vi "Ref Est.vi"(9 "touch":bool, 10 "IA State Input":T2) -> (1 "IA command":T1, 2 "IA State Output":T2)   [LabVIEW 2024, in "Referee.lvclass"]
uses:
  Referee.lvclass
  Vision_class/Old vision/SSL Detection Frame Simple Estimator Cameras VelCmd Folder/Core/AI Input.ctl
  Vision_class/Old vision/Controls/AI Robot.ctl
  Vision_class/Old vision/Controls/Functions Enum.ctl
  Controls/estimatives.ctl
  Vision_class/Old vision/Controls/AttackerStates.ctl
  Vision_class/Old vision/Controls/PathDests.ctl
  Vision_class/Old vision/Controls/PathDest.ctl
  Game_class/Navigation/VSSNavigation/VSSAttackerStates.ctl
  Robot_class/robotKickToStates.ctl
  Robot_class/roles.ctl
  <vilib>/Analysis/Matrix/Datatypes/RealMatrix.ctl
  Game_class/Navigation/driveMode.ctl
  Vision_class/Old vision/SSL Detection Frame Simple Estimator Cameras VelCmd Folder/Core/AI Ball.ctl
  Vision_class/Old vision/SSL Detection Frame Simple Estimator Cameras VelCmd Folder/Core/Field Size.ctl
  Vision_class/Old vision/SSL Detection Frame Simple Estimator Cameras VelCmd Folder/Core/AI Judge.ctl
  Communication_class/Paths/MessageAI_State Folder/Intel/Command Enum.ctl
  Vision_class/Old vision/SSL Detection Frame Simple Estimator Cameras VelCmd Folder/Util/Events/Events.ctl
  <vilib>/Analysis/Matrix/NI_Matrix.lvlib
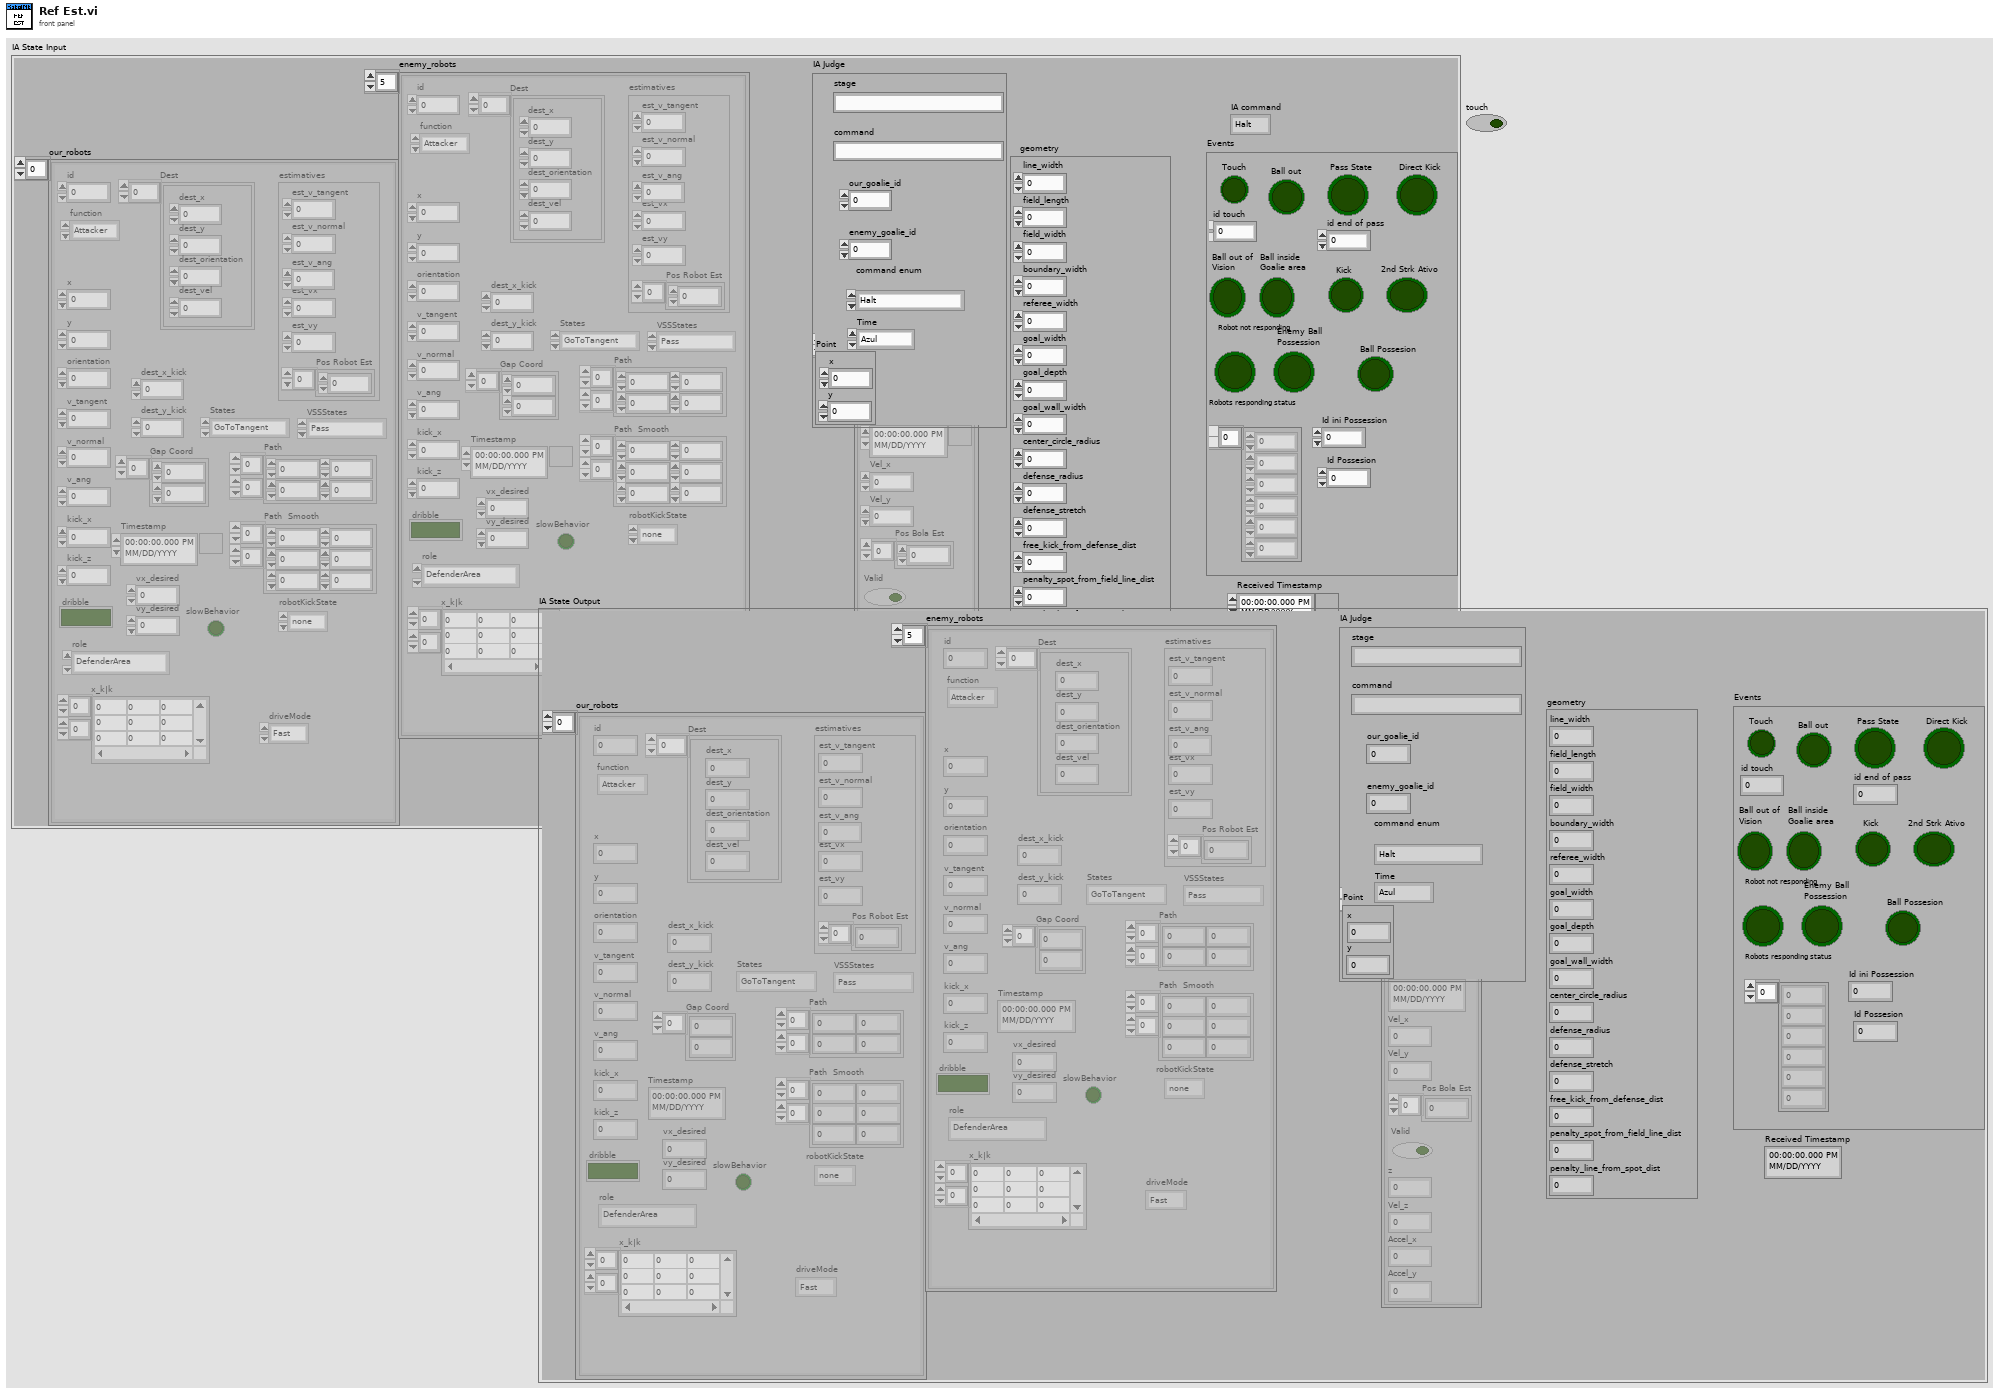
[diagram p1: front panel]
types:
  T1 = typedef "Command Enum.ctl" = enum16{"Halt", "Stop", "Force Start", "PKA Normal Start", "Prepare Kickoff Ally", "PKE Normal Start", "Prepare Kickoff Enemy", "Prepare Penalty Ally", "PPA Normal Start", "Prepare Penalty Enemy", "PPE Normal Start", "Direct Free Enemy", "Direct Free Ally", "Indirect Free Enemy", "Indirect Free Ally", "Timeout Enemy", "Timeout Ally", "Goal Enemy", "Goal Ally", "Ball Placement Enemy", "Ball Placement Ally", "Normal Half Time", "Extra Time Break", "Extra Half Time", "None", "Post Game", "S Normal Start"}
  T2 = typedef "AI Input.ctl" = cluster{"our_robots":T3[], "enemy_robots":T3[], "balls":T14[], "geometry":T15, "IA Judge":T16, "Received Timestamp":timestamp, "Events":T17}
  T3 = typedef "AI Robot.ctl" = cluster{"id":u32, "function":T4, "x":dbl, "y":dbl, "orientation":dbl, "v_tangent":dbl, "v_normal":dbl, "v_ang":dbl, "kick_x":dbl, "kick_z":dbl, "dribble":bool, "Timestamp":timestamp, "estimatives":T5, "dest_x_kick":dbl, "dest_y_kick":dbl, "Gap Coord":dbl[], "States":T6, "Path ":dbl[][], "Path  Smooth":dbl[][], "Dest":T7, "vx_desired":dbl, "vy_desired":dbl, "slowBehavior":bool, "VSSStates":T9, "robotKickState":T10, "role":T11, "x_k|k":T12, "driveMode":T13}
  T4 = typedef "Functions Enum.ctl" = enum16{"2nd Striker", "Attacker", "Goalie", "Defender", "Striker", "Goto 0", "Dummy", "Kicker", "ZigZag 0", "ZigZag 1", "ZigZag 2", "ZigZag 3", "ZigZag 4", "ZigZag 5", "ZigZag 6", "ZigZag 7", "ZigZag 8", ""}
  T5 = typedef "estimatives.ctl" = cluster{"est_v_tangent":dbl, "est_v_normal":dbl, "est_vx":dbl, "est_vy":dbl, "Pos Robot Est":dbl[], "est_v_ang":dbl}
  T6 = typedef "AttackerStates.ctl" = enum16{"Pass", "GoToTangent", "BallGetting", "GoToKick", ""}
  T7 = typedef "PathDests.ctl" = T8[]
  T8 = typedef "PathDest.ctl" = cluster{"dest_x":dbl, "dest_y":dbl, "dest_orientation":dbl, "dest_vel":dbl}
  T9 = typedef "VSSAttackerStates.ctl" = enum16{"Pass", "GoToTangent", "BallGetting", "GoToKick", "Rotate anti-clockwise", "Rotate Clockwise", ""}
  T10 = typedef "robotKickToStates.ctl" = enum16{"shootFromDirect", "avoidCollideBall", "goToBackBall", "none", "walk", "turn", "turnAntiClockWise", "turnClockwise", "oldKickToShoot", "oldKickToGoToBackBall", "shoot"}
  T11 = typedef "roles.ctl" = enum16{"SimpleBallPlacement", "BallPlacementAllyPasser", "BallPlacementAllyReceiver", "BallPlacementEnemy", "5Robots5th", "PassBestReceiver", "5Robots4th", "5Robots3rd", "5Robots2nd", "5Robots1st", "PassBestRobot", "WaitPass", "ABCThirdKicker", "ABCFirstKicker", "ABCSecondKicker", "Tabler", "TableFinalizer", "PrepareRollToPassRoller", "PrepareRollToPassReceiver", "SimplePassRoll", "SimplePassRollReceiver", "PenaltyDefense", "PreparePassReceiver 2", "PreparePassReceiver 1", "PassObserver", "Timeout", "Goto", "ZigZag", "None", "BallOutOfField", "DefenderArea", "Duelist", "AttackerStop", "FollowAttacker", "KeeperRole", "KickPenalty", "AttackerAimGoal", "AttackerBlock", "Marker", "Halt", "Shoot", "PassKicker", "PassReceiver", "TestRole", "PenaltyAttacker"}
  T12 = typedef "NI_Matrix.lvlib/RealMatrix.ctl" = dbl[][]
  T13 = typedef "driveMode.ctl" = enum16{"Fast", "SafeDrive"}
  T14 = typedef "AI Ball.ctl" = cluster{"x":dbl, "y":dbl, "timestamp":timestamp, "Vel_x":dbl, "Vel_y":dbl, "Pos Bola Est":dbl[], "Valid":bool, "z":dbl, "Vel_z":dbl, "Accel_x":dbl, "Accel_y":dbl}
  T15 = typedef "Field Size.ctl" = cluster{"line_width":u32, "field_length":u32, "field_width":u32, "boundary_width":u32, "referee_width":u32, "goal_width":u32, "goal_depth":u32, "goal_wall_width":u32, "center_circle_radius":u32, "defense_radius":u32, "defense_stretch":u32, "free_kick_from_defense_dist":u32, "penalty_spot_from_field_line_dist":u32, "penalty_line_from_spot_dist":u32}
  T16 = typedef "AI Judge.ctl" = cluster{"stage":string, "command":string, "our_goalie_id":dbl, "enemy_goalie_id":dbl, "command enum":T1, "Time":enum16{"Azul", "Amarelo"}, "Point":cluster{"x":sgl, "y":sgl}}
  T17 = typedef "Events.ctl" = cluster{"Touch":bool, "Ball out":bool, "id touch":dbl, "Ball out of \nVision":bool, "Ball inside \nGoalie area":bool, "Robot not responding":bool, "Robots responding status":dbl[], "Enemy Ball \nPossession":bool, "Pass State":bool, "id end of pass":dbl, "Kick":bool, "Id ini Possession":dbl, "Ball Possesion":bool, "Id Possesion":dbl, "Direct Kick":bool, "2nd Strk Ativo":bool}
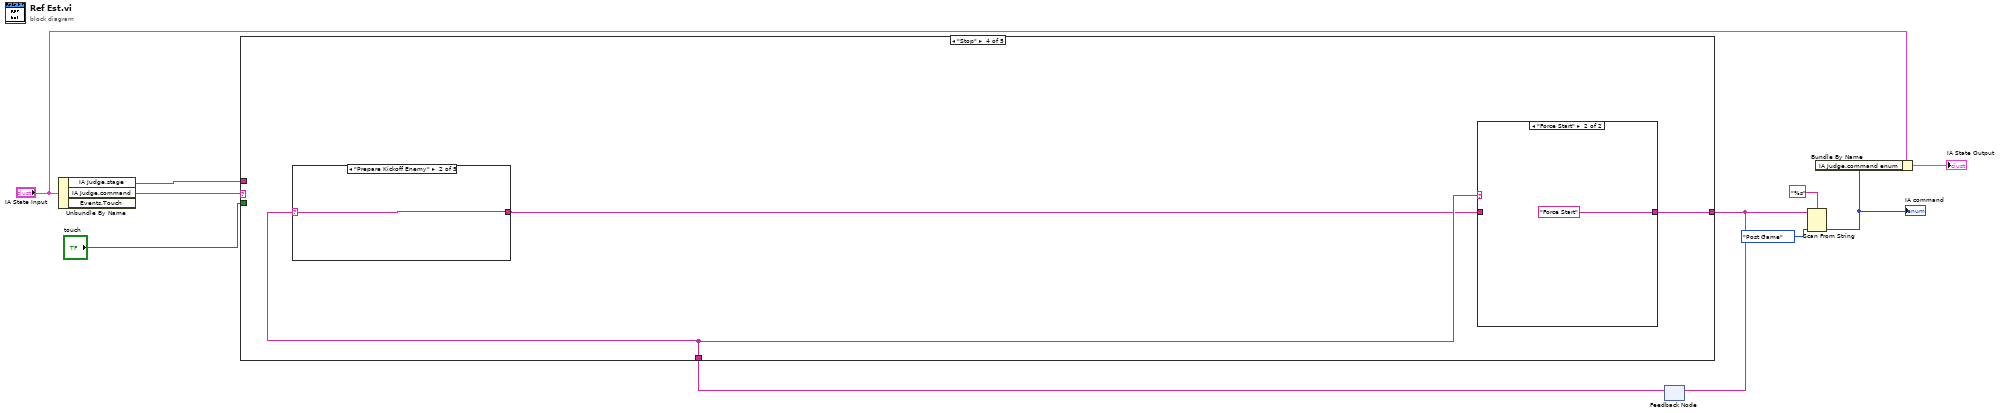
[diagram p0: block diagram]
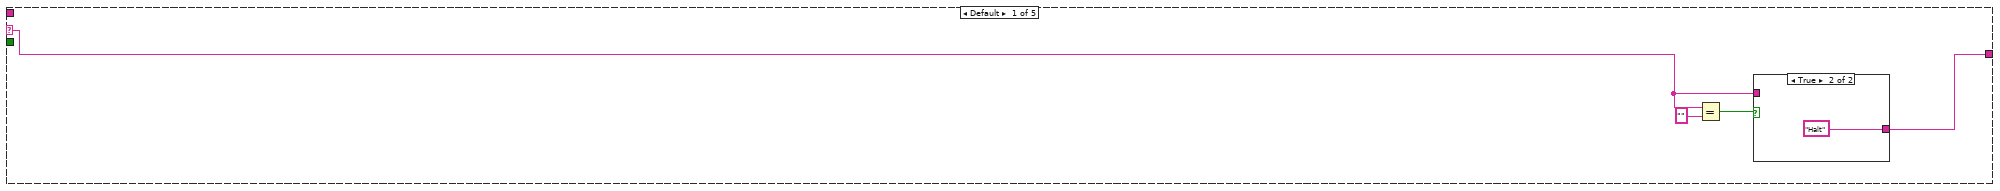
[diagram p2: hidden frame]
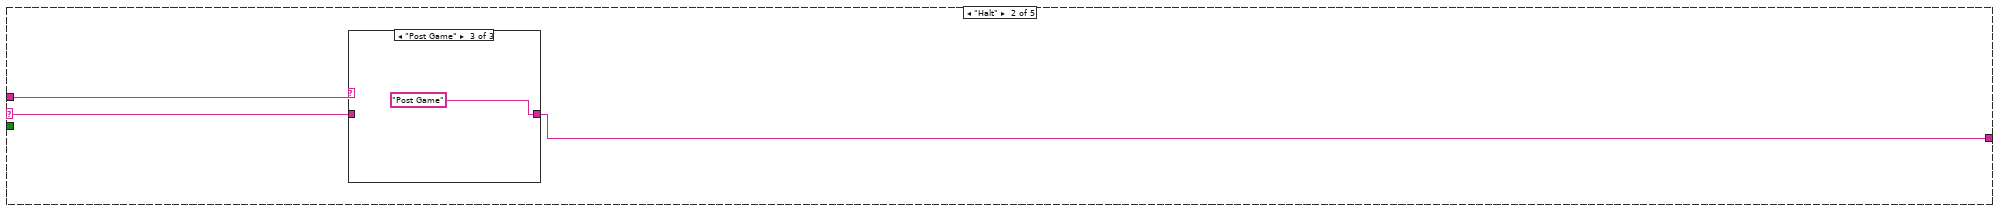
[diagram p4: hidden frame]
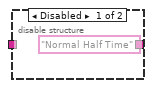
[diagram p7: hidden frame]
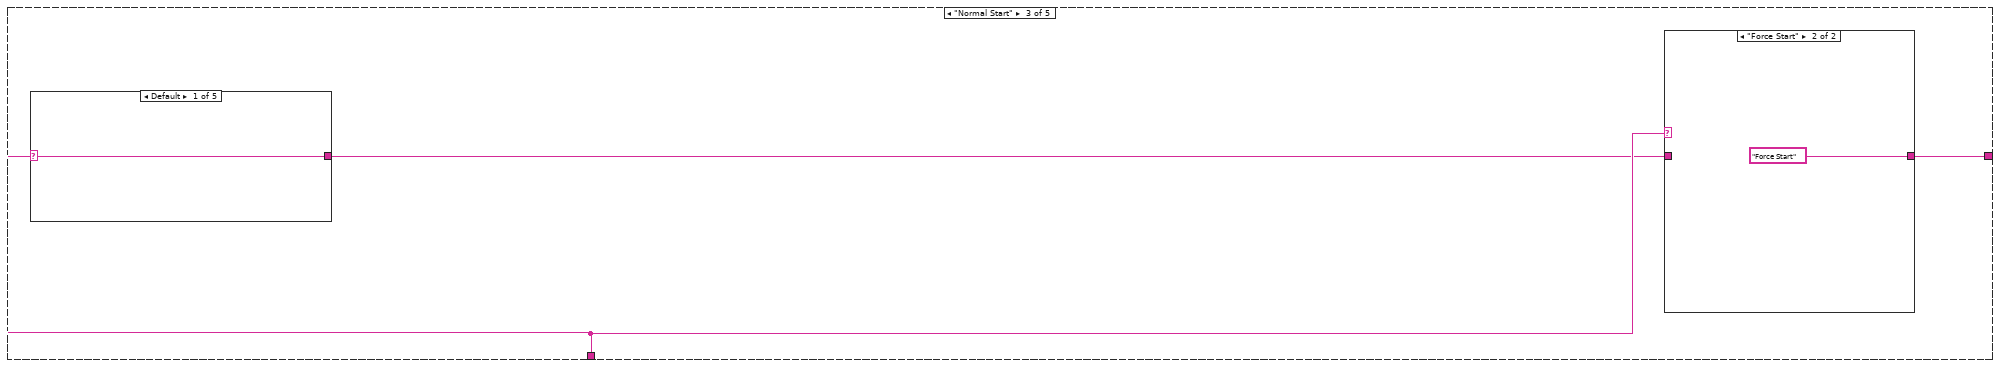
[diagram p8: hidden frame]
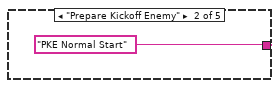
[diagram p10: hidden frame]
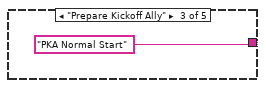
[diagram p11: hidden frame]
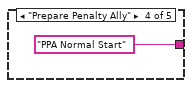
[diagram p12: hidden frame]
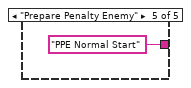
[diagram p13: hidden frame]
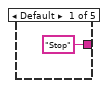
[diagram p15: hidden frame]
diagram:
  n1 = Unbundle By Name("IA State Input") -> ("IA Judge.stage"=w3:string, "IA Judge.command"=w10:string)  [unwired: 1 out]
  n2 = feedback #1() -> (w5:string)  [unwired: 1 in]
  n3 = case shown="\"Stop\"" w10 {
    selector: w10 -> [w11 w18 _ _ w46]
    tunnel: [w13 w17 w28 w38 w46] -> w4
    tunnel: w5 -> [_ _ w27 w37 _]
    tunnel: "touch" -> [_ _ _ _ _]
    tunnel: w3 -> [_ w19 _ _ _]
    frame Default {
      n4 = Equal?(x=w11, y="") -> (x = y?=w12:bool)
      n5 = case shown="True" w12 {
        tunnel: [w15 "Halt" ("y")] -> w13
        tunnel: w11 -> [w15 _]
        frame False {
        }
        frame True {
        }
      }
    }
    frame "Halt" {
      n6 = case shown="\"Post Game\"" w19 {
        tunnel: [w20 w22 "Post Game"] -> w17
        tunnel: w18 -> [w20 w21 _]
        frame Default {
        }
        frame "Normal Half Time" {
          n7 = disable-structure shown="Enabled" {
            disable-tunnel: ["Normal Half Time" w24] -> w22
            disable-tunnel: w21 -> [_ w24]
            frame Disabled {
            }
            frame Enabled {
            }
          }
        }
        frame "Post Game" {
        }
      }
    }
    frame "Normal Start" {
      n8 = case shown="Default" w27 {
        selector: w27 -> [w31 _ _ _ _]
        tunnel: [w31 "PKE Normal Start" "PKA Normal Start" "PPA Normal Start" "PPE Normal Start"] -> w26
        frame Default {
        }
        frame "Prepare Kickoff Enemy" {
        }
        frame "Prepare Kickoff Ally" {
        }
        frame "Prepare Penalty Ally" {
        }
        frame "Prepare Penalty Enemy" {
        }
      }
      n9 = case shown="\"Force Start\"" w27 {
        tunnel: [w29 "Force Start"] -> w28
        tunnel: w26 -> [w29 _]
        frame Default {
        }
        frame "Force Start" {
        }
      }
    }
    frame "Stop" {
      n10 = case shown="\"Prepare Kickoff Enemy\"" w37 {
        selector: w37 -> [_ w42 w43 w44 w45]
        tunnel: ["Stop" w42 w43 w44 w45] -> w36
        frame Default {
        }
        frame "Prepare Kickoff Enemy" {
        }
        frame "Prepare Kickoff Ally" {
        }
        frame "Prepare Penalty Ally" {
        }
        frame "Prepare Penalty Enemy" {
        }
      }
      n11 = case shown="\"Force Start\"" w37 {
        tunnel: [w39 "Force Start"] -> w38
        tunnel: w36 -> [w39 _]
        frame Default {
        }
        frame "Force Start" {
        }
      }
    }
    frame "Direct Free Enemy", "Indirect Free Enemy" {
    }
  }
  n12 = feedback-in #1(w4) -> ()
  n13 = Scan From String(format string="%s", input string=w4, default 1=Command_Enum."Post Game" ("command\nenum")) -> (output 1=w7:T1)  [unwired: 2 in, 3 out]
  "IA command" <- w7
  n14 = Bundle By Name(cluster="IA State Input", "IA Judge.command enum"=w7) -> (→"IA State Output":T2)
